vi "911 Vehicle Approach.vi"(3 "Cycle State In":T1) -> (0 "Cycle State Out":T1)   [LabVIEW 2020]
uses:
  Reset.ctl
  Cycle Status.ctl
  Cycle Enum.ctl
  Grade Gate.ctl
  Global Indicators.vi
panel:
  out "Cycle Status":T2
  in  "Reset":T3
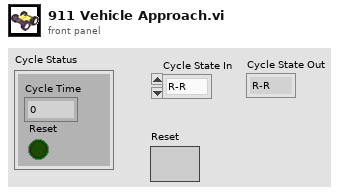
[diagram p1: front panel]
types:
  T1 = typedef "Cycle Enum.ctl" = enum16{"R-R", "NS Left G", "NS Left Y", "NS Straight G", "NS Straight Y", "r-r", "WE Left G", "WE Left Y", "WE Straight G", "WE Straight Y", "N All G", "S All G", "W All G", "E All G", "Gate Up", "Gate Mid", "Blink 1", "End Train", "Blink 2"}
  T2 = typedef "Cycle Status.ctl" = cluster{"Cycle Time":dbl, "Reset":bool}
  T3 = typedef "Reset.ctl" = bool
  T4 = typedef "Grade Gate.ctl" = cluster{"UP 2":bool, "Pivot":bool, "UP 3":bool, "UP 4":bool, "UP 5":bool, "UP 6":bool, "DOWN 2":bool, "DOWN 3":bool, "DOWN 4":bool, "DOWN 5":bool, "DOWN 6":bool, "DOWN 7":bool, "DOWN 8":bool, "SIDE 2":bool, "SIDE 3":bool, "SIDE 4":bool, "SIDE 5":bool, "Blinky 2":bool, "Blinky 1":bool}
  T5 = typedef "Traffic Signal.ctl" = cluster{"Red Light":bool, "Yellow Light":bool, "Green Light":bool, "Yellow Turn":bool, "Green Turn":bool}
  T6 = typedef "PedX Signal.ctl" = cluster{"PedX Walk":bool, "PedX Stop":bool}
  T7 = enum16{"R-R", "NS Left G", "NS Left Y", "NS Straight G", "NS Straight Y", "r-r", "WE Left G", "WE Left Y", "WE Straight G", "WE Straight Y"}
  T8 = enum16{"R-R", "NS Left G", "NS Left Y", "NS Straight G", "NS Straight Y"}
  T9 = cluster{"North":bool, "South":bool, "West":bool, "East":bool}
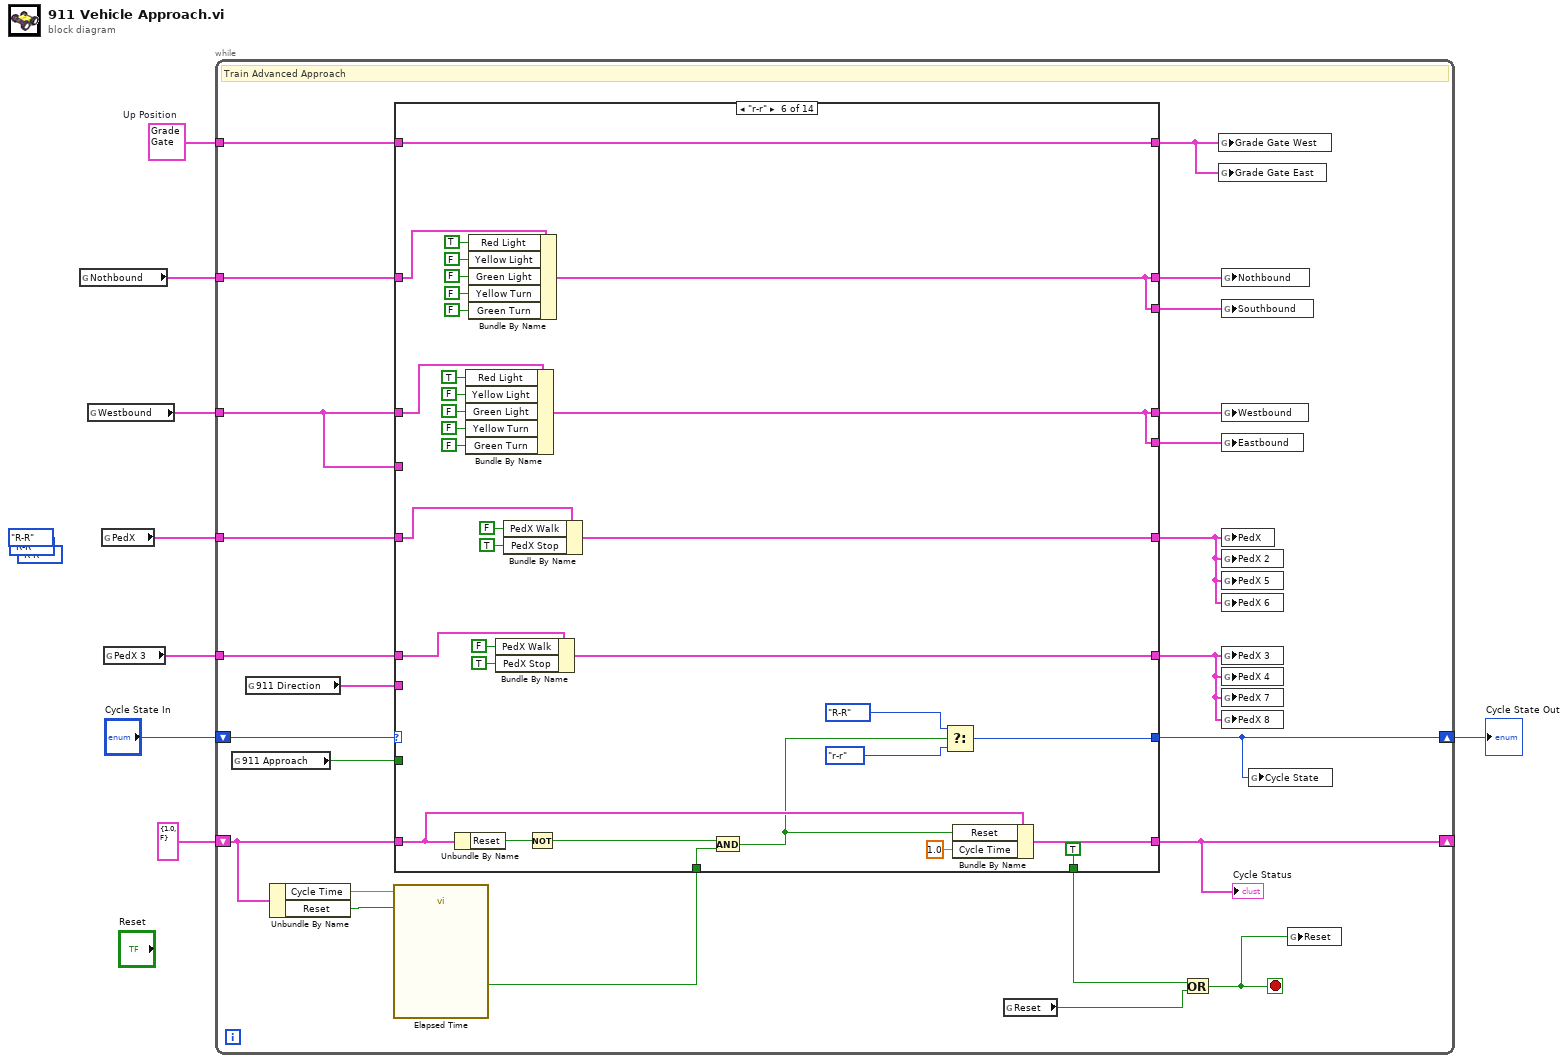
[diagram p0: block diagram]
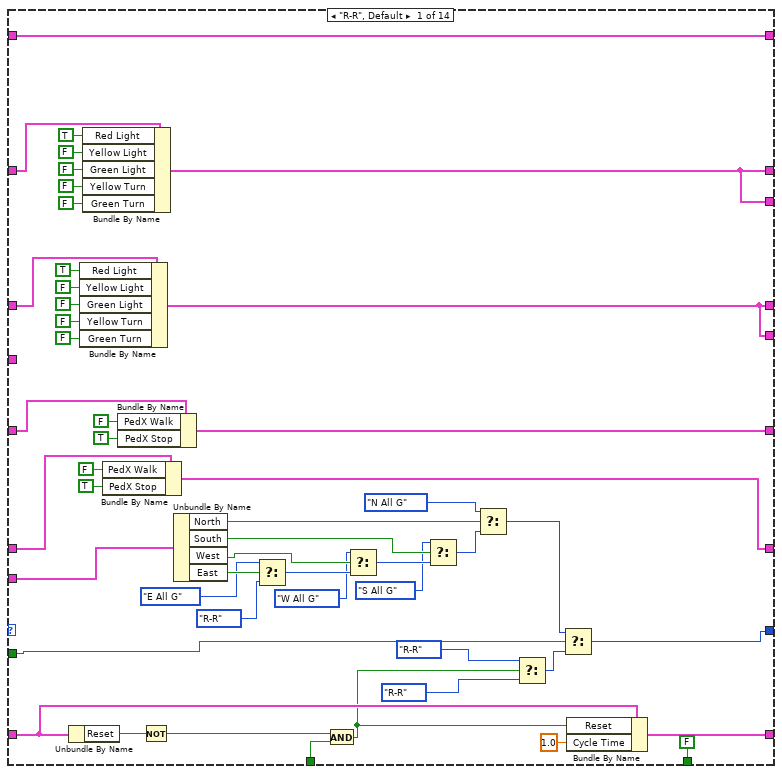
[diagram p2: hidden frame]
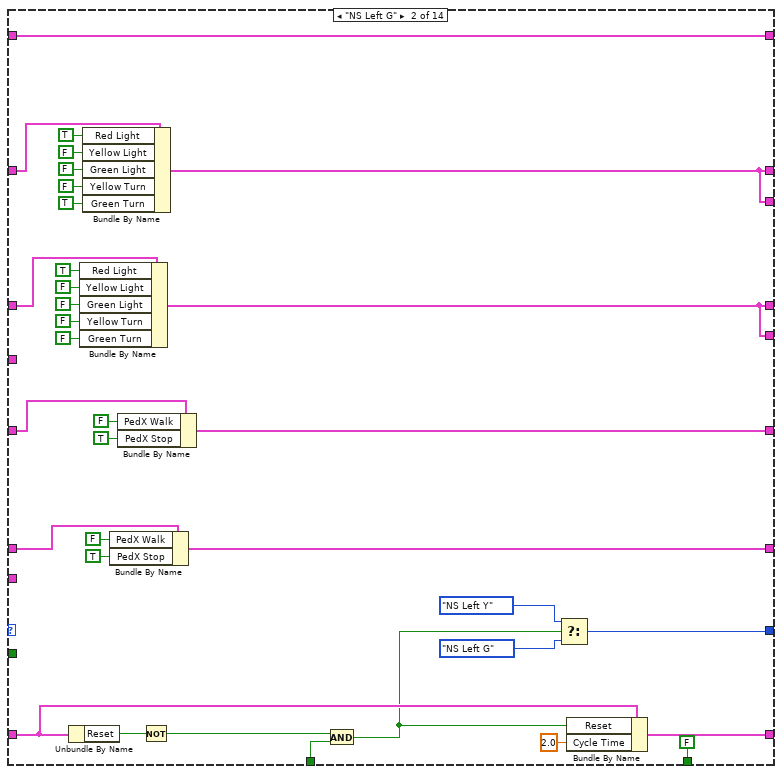
[diagram p3: hidden frame]
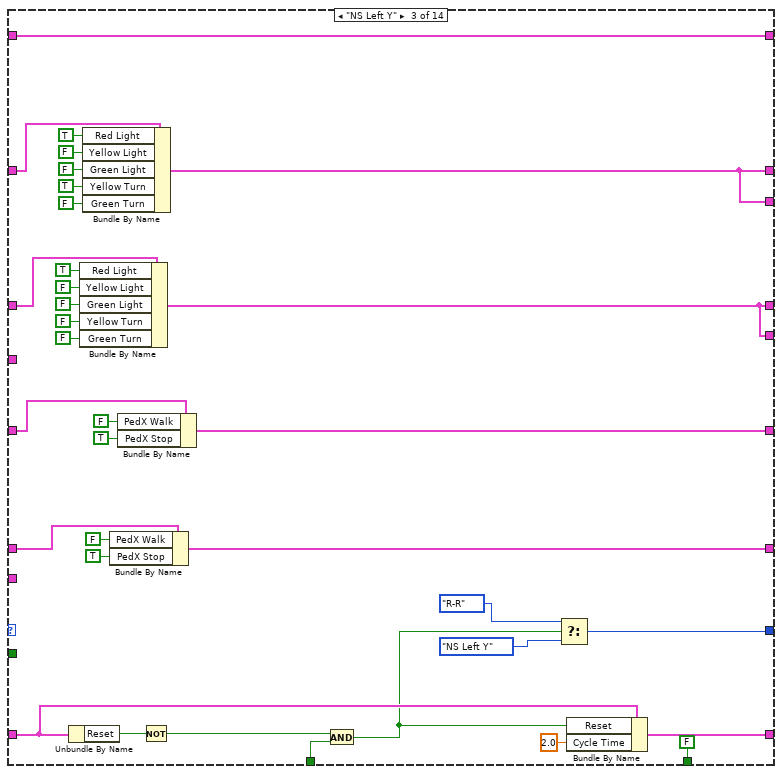
[diagram p4: hidden frame]
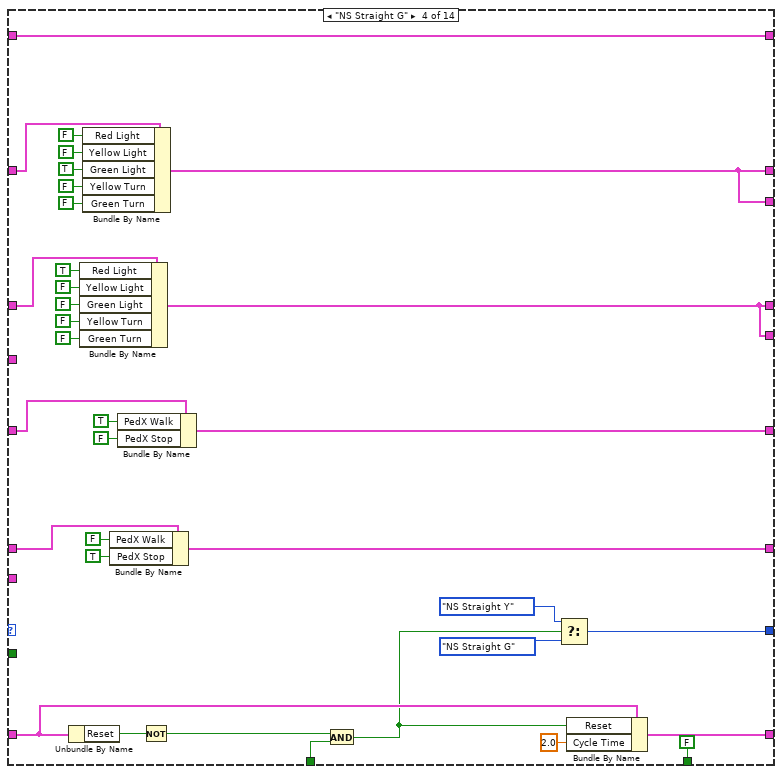
[diagram p5: hidden frame]
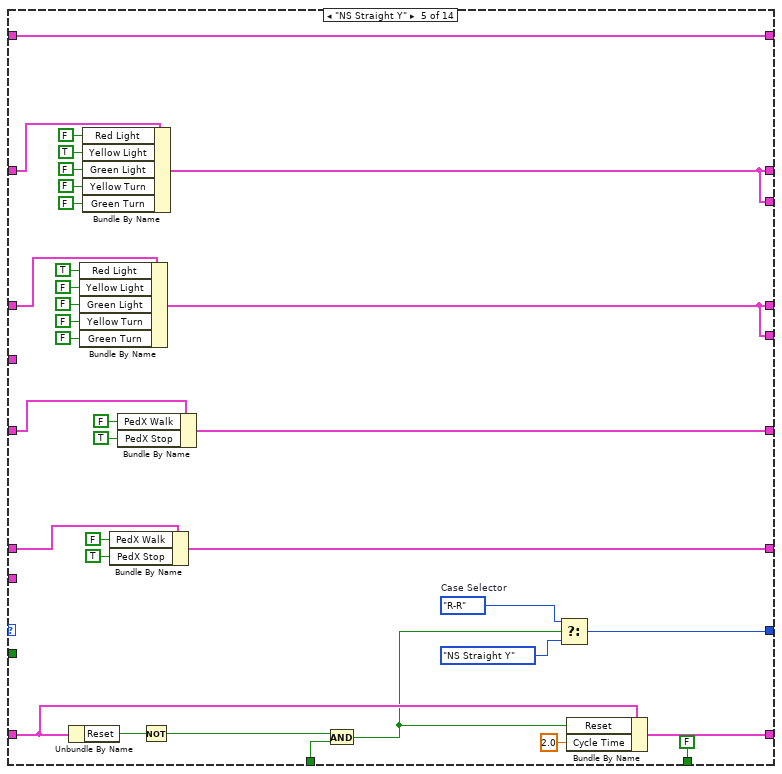
[diagram p6: hidden frame]
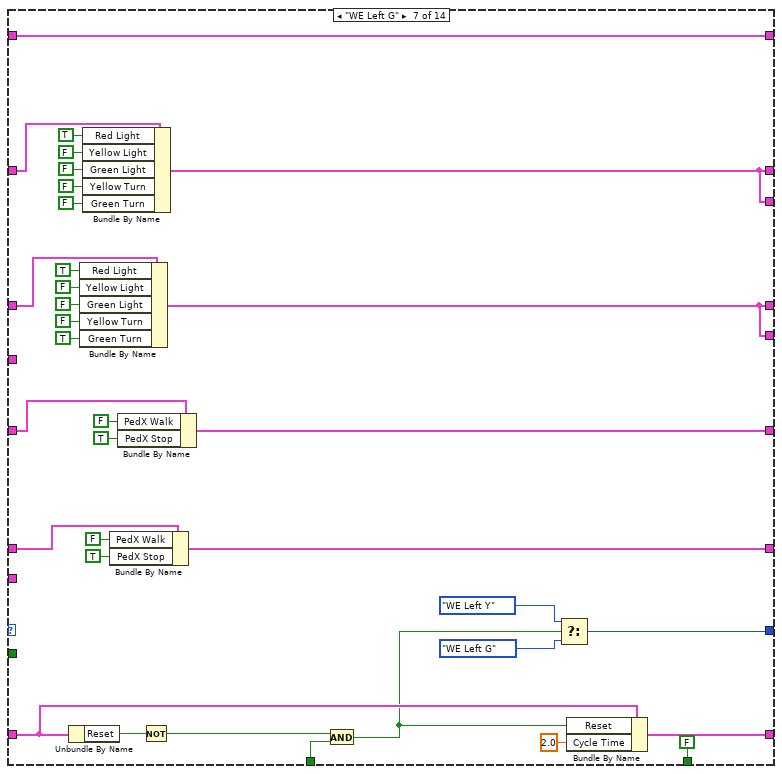
[diagram p7: hidden frame]
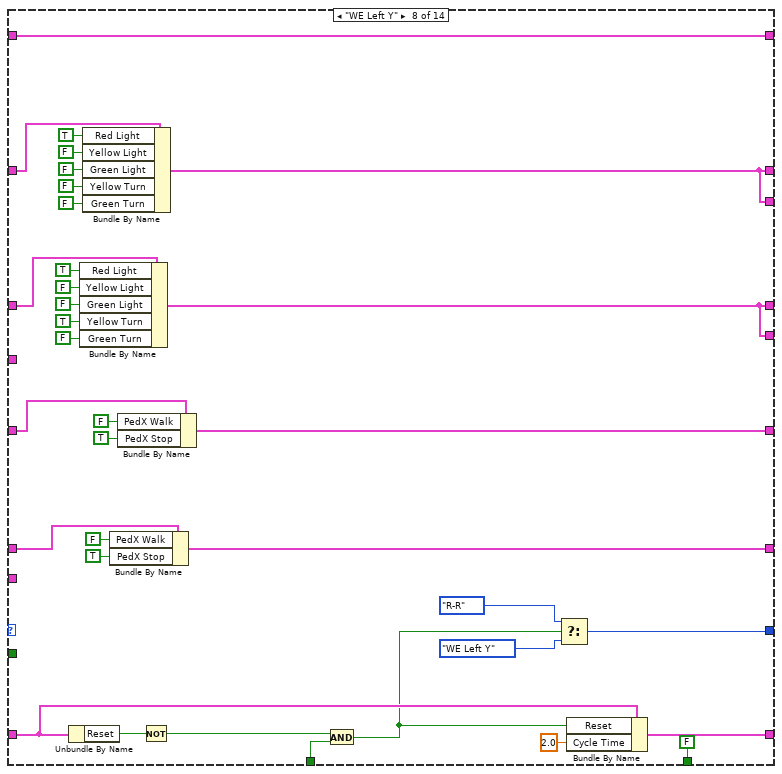
[diagram p8: hidden frame]
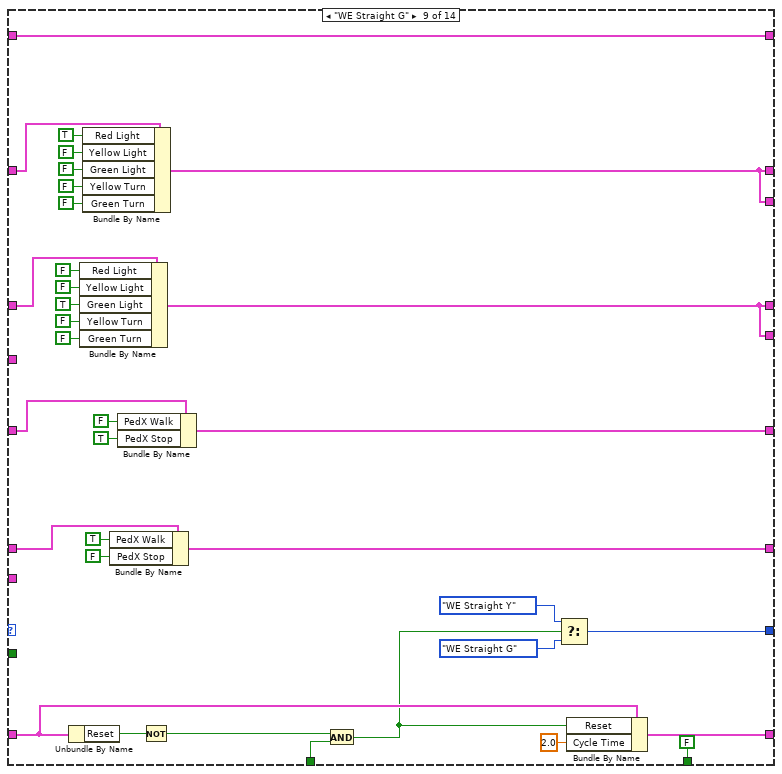
[diagram p9: hidden frame]
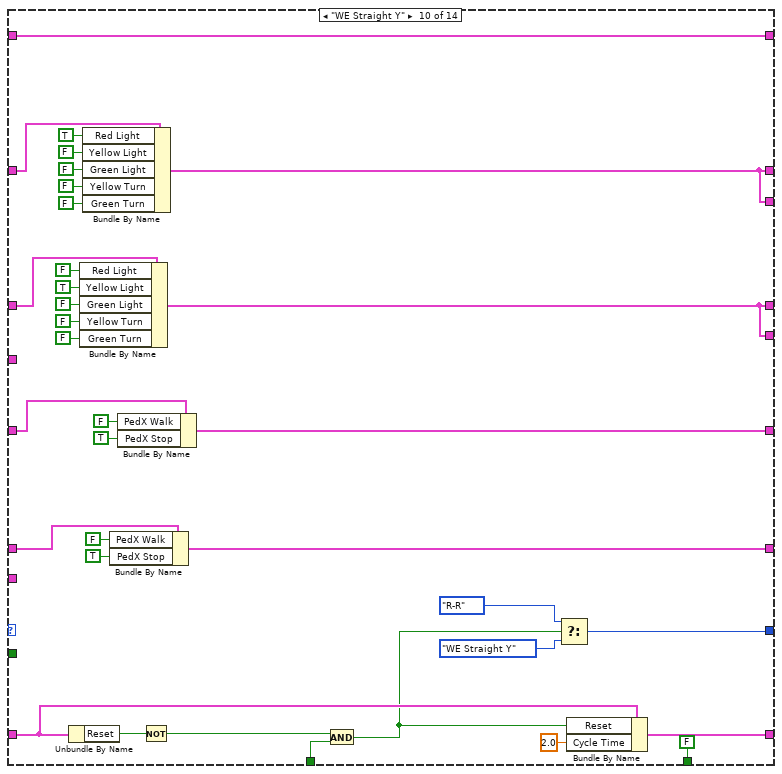
[diagram p10: hidden frame]
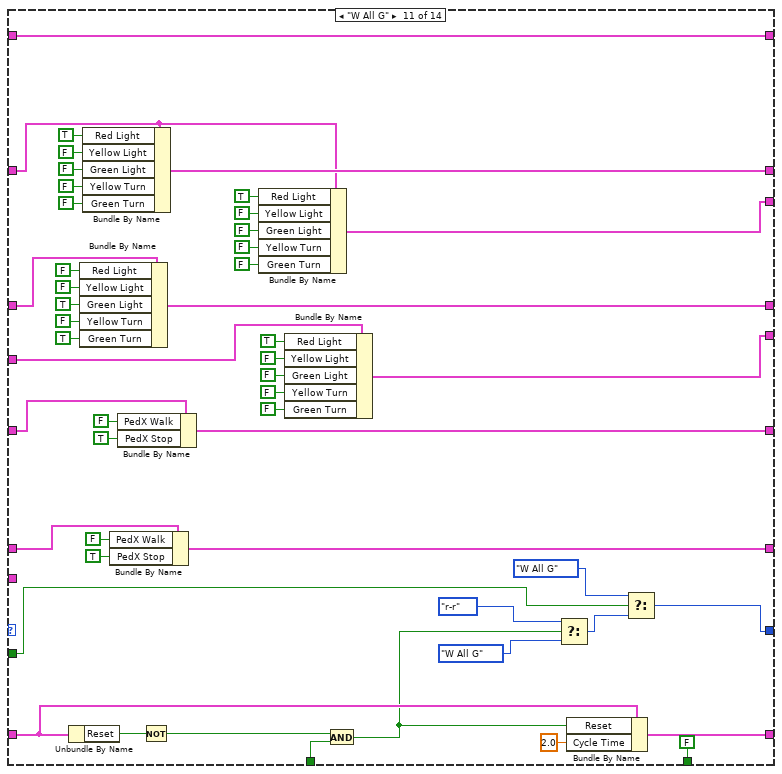
[diagram p11: hidden frame]
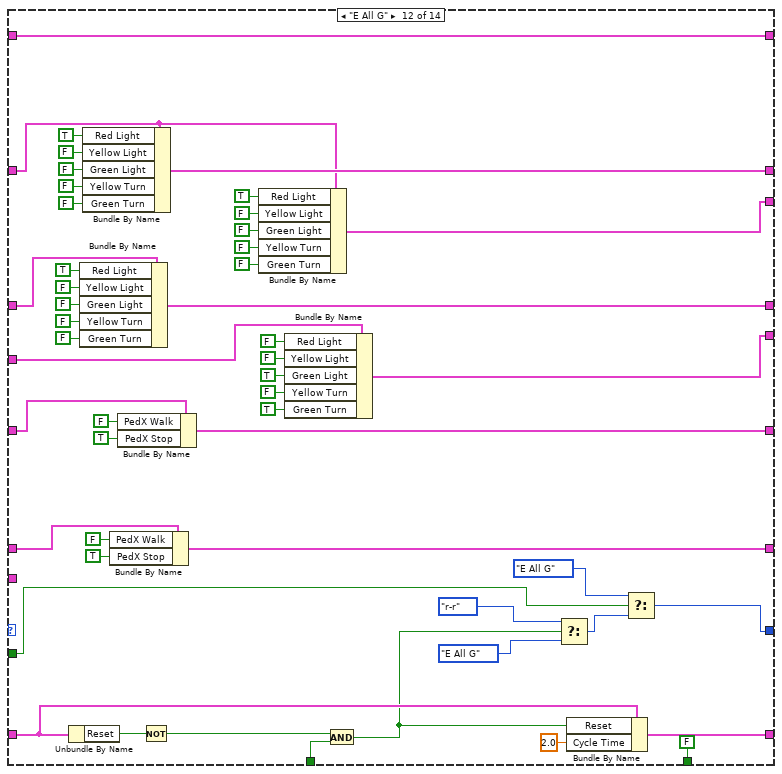
[diagram p12: hidden frame]
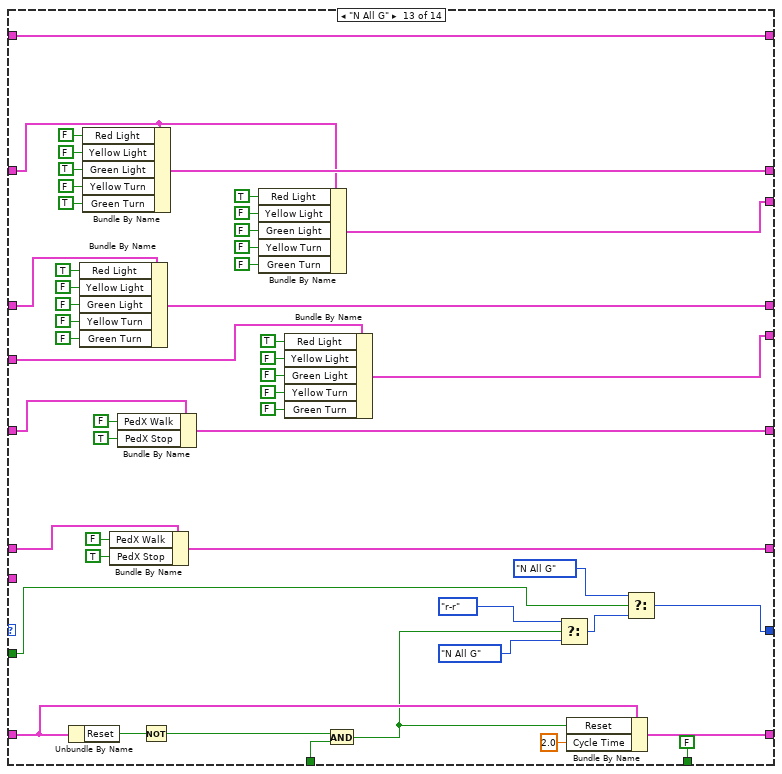
[diagram p13: hidden frame]
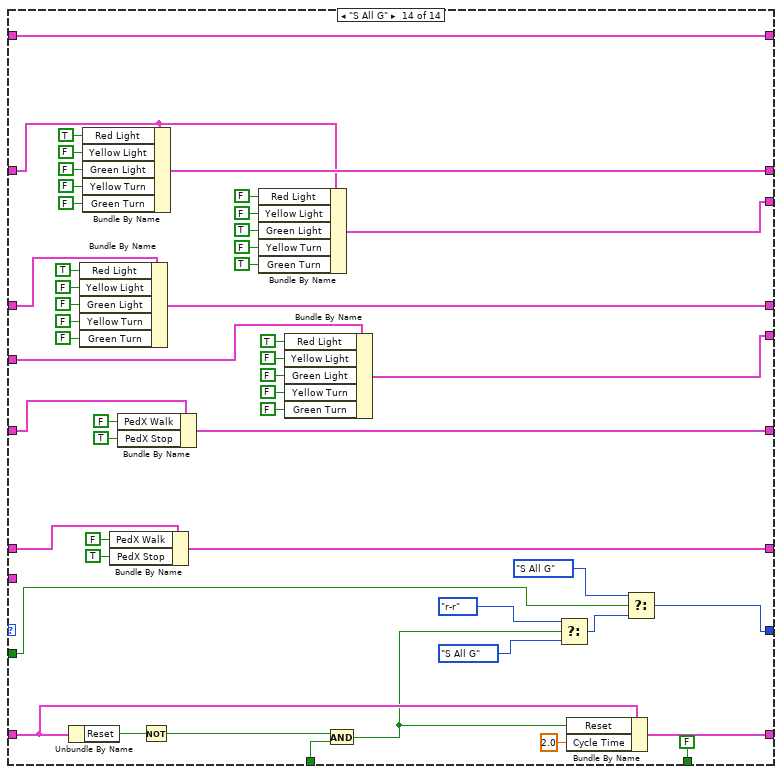
[diagram p14: hidden frame]
diagram:
  (unwired) Cycle_Enum."R-R" ("Cycle State In")
  (unwired) Cycle_Enum."R-R" ("Cycle State In")
  (unwired) Cycle_Enum."R-R" ("Cycle State In")
  w8 = T4 {"UP 2"=FALSE, "Pivot"=FALSE, "UP 3"=TRUE, "UP 4"=FALSE, "UP 5"=FALSE, "UP 6"=FALSE, "DOWN 2"=FALSE, "DOWN 3"=FALSE, "DOWN 4"=FALSE, "DOWN 5"=FALSE, "DOWN 6"=FALSE, "DOWN 7"=FALSE, "DOWN 8"=FALSE, "SIDE 2"=FALSE, "SIDE 3"=FALSE, "SIDE 4"=FALSE, "SIDE 5"=FALSE, "Blinky 2"=FALSE, "Blinky 1"=FALSE}  # Up Position
  n1 = global read "Global Indicators.vi" "Nothbound"() -> (w6:T5)
  n2 = global read "Global Indicators.vi" "Westbound"() -> (w5:T5)
  n3 = global read "Global Indicators.vi" "PedX"() -> (w4:T6)
  n4 = global read "Global Indicators.vi" "PedX 3"() -> (w3:T6)
  n5 = while {
    shift-right: [w17] -> w1
    shift-left: "Cycle State In" -> [w19]
    tunnel: w8 -> [w28]
    tunnel: w5 -> [w16]
    tunnel: w6 -> [w27]
    tunnel: w4 -> [w26]
    tunnel: w3 -> [w25]
    shift-right: [w18] -> _
    shift-left: T2 {"Cycle Time"=1.0, "Reset"=FALSE} ("Cycle Status") -> [w24]
    stop <- w11 stop-if-true
    # "Train Advanced Approach"
    n6 = global read "Global Indicators.vi" "911 Approach"() -> (w12:bool)
    n7 = global read "Global Indicators.vi" "911 Direction"() -> (w10:T9)
    n8 = Unbundle By Name(w24) -> ("Cycle Time"=w32:dbl, "Reset"=w31:bool)
    n9 = call "Elapsed Time"("Time Target (s)"=w32, "Reset"=w31) -> ("Time has Elapsed"=w30:bool)  [unwired: 10 in, 7 out]
    n10 = case shown="\"r-r\"" w19 {
      tunnel: [w82 w116 w150 w184 w218 w252 w286 w320 w354 w388 w438 w488 w538 w588] -> w29
      tunnel: w28 -> [w82 w116 w150 w184 w218 w252 w286 w320 w354 w388 w438 w488 w538 w588]
      tunnel: [w33 w83 w117 w151 w185 w219 w253 w287 w321 w355 w432 w482 w532 w582] -> w23
      tunnel: w27 -> [w81 w115 w149 w183 w217 w251 w285 w319 w353 w387 w395 w445 w495 w545]
      tunnel: [w53 w85 w119 w153 w187 w221 w255 w289 w323 w357 w419 w469 w519 w569] -> w22
      tunnel: w16 -> [w64 w97 w130 w163 w199 w233 w267 w301 w335 w369 w420 w470 w520 w570]
      tunnel: [w72 w106 w140 w174 w208 w242 w276 w310 w344 w378 w428 w478 w528 w578] -> w21
      tunnel: w26 -> [w75 w109 w143 w177 w211 w245 w279 w313 w347 w381 w431 w481 w531 w581]
      tunnel: w25 -> [w55 w88 w121 w154 w190 w224 w258 w292 w326 w360 w410 w460 w510 w560]
      tunnel: [w56 w89 w122 w155 w191 w225 w259 w293 w327 w361 w411 w461 w511 w561] -> w20
      tunnel: [w68 w101 w134 w167 w203 w237 w271 w305 w339 w373 w424 w474 w524 w574] -> w18
      tunnel: w24 -> [w67 w100 w133 w166 w202 w236 w270 w304 w338 w372 w423 w473 w523 w573]
      tunnel: [w49 w102 w136 w170 w204 w238 w272 w306 w340 w374 w396 w446 w496 w546] -> w17
      tunnel: w30 -> [w69 w103 w137 w171 w205 w239 w273 w307 w341 w375 w425 w475 w525 w575]
      tunnel: w16 -> [_ _ _ _ _ _ _ _ _ _ w409 w459 w509 w559]
      tunnel: [w53 w85 w119 w153 w187 w221 w255 w289 w323 w357 w403 w453 w503 w553] -> w15
      tunnel: w12 -> [w48 _ _ _ _ _ _ _ _ _ w399 w449 w499 w549]
      tunnel: [FALSE FALSE FALSE FALSE FALSE TRUE FALSE FALSE FALSE FALSE FALSE FALSE FALSE FALSE] -> w13
      tunnel: w10 -> [w47 _ _ _ _ _ _ _ _ _ _ _ _ _]
      tunnel: [w33 w83 w117 w151 w185 w219 w253 w287 w321 w355 w389 w439 w489 w539] -> w9
      frame "R-R", Default {
        n11 = Unbundle By Name(w67) -> ("Reset"=w71:bool)
        n12 = Bundle By Name(cluster=w64, "Red Light"=TRUE, "Yellow Light"=FALSE, "Green Light"=FALSE, "Yellow Turn"=FALSE, "Green Turn"=FALSE) -> (w53:T5)
        n13 = Bundle By Name(cluster=w81, "Red Light"=TRUE, "Yellow Light"=FALSE, "Green Light"=FALSE, "Yellow Turn"=FALSE, "Green Turn"=FALSE) -> (w33:T5)
        n14 = Bundle By Name(cluster=w55, "PedX Walk"=FALSE, "PedX Stop"=TRUE) -> (w56:T6)
        n15 = Bundle By Name(cluster=w75, "PedX Walk"=FALSE, "PedX Stop"=TRUE) -> (w72:T6)
        n16 = Not(x=w71) -> (.not. x?=w70:bool)
        n17 = Unbundle By Name(w47) -> ("North"=w46:bool, "South"=w38:bool, "West"=w42:bool, "East"=w45:bool)
        n18 = Select(t=Cycle_Enum."E All G" ("Cycle State In"), s=w45, f=Cycle_Enum."R-R" ("Cycle State In")) -> (s? t:f=w41:T1)
        n19 = And(x=w70, y=w69) -> (x .and. y?=w66:bool)
        n20 = Select(t=Cycle_Enum."W All G" ("Cycle State In"), s=w42, f=w41) -> (s? t:f=w39:T1)
        n21 = Select(t=Cycle_Enum."S All G" ("Cycle State In"), s=w38, f=w39) -> (s? t:f=w36:T1)
        n22 = Select(t=Cycle_Enum."N All G" ("Cycle State In"), s=w46, f=w36) -> (s? t:f=w34:T1)
        n23 = Select(t=Cycle_Enum."R-R" ("Cycle State In"), s=w66, f=Cycle_Enum."R-R" ("Cycle State In")) -> (s? t:f=w50:T1)
        n24 = Select(t=w34, s=w48, f=w50) -> (s? t:f=w49:T1)
        n25 = Bundle By Name(cluster=w67, "Reset"=w66, "Cycle Time"=1.0) -> (w68:T2)
      }
      frame "NS Left G" {
        n26 = Unbundle By Name(w100) -> ("Reset"=w105:bool)
        n27 = Bundle By Name(cluster=w97, "Red Light"=TRUE, "Yellow Light"=FALSE, "Green Light"=FALSE, "Yellow Turn"=FALSE, "Green Turn"=FALSE) -> (w85:T5)
        n28 = Bundle By Name(cluster=w115, "Red Light"=TRUE, "Yellow Light"=FALSE, "Green Light"=FALSE, "Yellow Turn"=FALSE, "Green Turn"=TRUE) -> (w83:T5)
        n29 = Bundle By Name(cluster=w88, "PedX Walk"=FALSE, "PedX Stop"=TRUE) -> (w89:T6)
        n30 = Bundle By Name(cluster=w109, "PedX Walk"=FALSE, "PedX Stop"=TRUE) -> (w106:T6)
        n31 = Not(x=w105) -> (.not. x?=w104:bool)
        n32 = And(x=w104, y=w103) -> (x .and. y?=w99:bool)
        n33 = Select(t=T7."NS Left Y" ("Case Selector"), s=w99, f=T7."NS Left G" ("Case Selector")) -> (s? t:f=w102:T7)
        n34 = Bundle By Name(cluster=w100, "Reset"=w99, "Cycle Time"=2.0) -> (w101:T2)
      }
      frame "NS Left Y" {
        n35 = Unbundle By Name(w133) -> ("Reset"=w139:bool)
        n36 = Bundle By Name(cluster=w130, "Red Light"=TRUE, "Yellow Light"=FALSE, "Green Light"=FALSE, "Yellow Turn"=FALSE, "Green Turn"=FALSE) -> (w119:T5)
        n37 = Bundle By Name(cluster=w149, "Red Light"=TRUE, "Yellow Light"=FALSE, "Green Light"=FALSE, "Yellow Turn"=TRUE, "Green Turn"=FALSE) -> (w117:T5)
        n38 = Bundle By Name(cluster=w121, "PedX Walk"=FALSE, "PedX Stop"=TRUE) -> (w122:T6)
        n39 = Bundle By Name(cluster=w143, "PedX Walk"=FALSE, "PedX Stop"=TRUE) -> (w140:T6)
        n40 = Not(x=w139) -> (.not. x?=w138:bool)
        n41 = And(x=w138, y=w137) -> (x .and. y?=w132:bool)
        n42 = Select(t=Cycle_Enum."R-R" ("Cycle State In"), s=w132, f=T8."NS Left Y" ("Case Selector")) -> (s? t:f=w136:T1)
        n43 = Bundle By Name(cluster=w133, "Reset"=w132, "Cycle Time"=2.0) -> (w134:T2)
      }
      frame "NS Straight G" {
        n44 = Unbundle By Name(w166) -> ("Reset"=w173:bool)
        n45 = Bundle By Name(cluster=w163, "Red Light"=TRUE, "Yellow Light"=FALSE, "Green Light"=FALSE, "Yellow Turn"=FALSE, "Green Turn"=FALSE) -> (w153:T5)
        n46 = Bundle By Name(cluster=w183, "Red Light"=FALSE, "Yellow Light"=FALSE, "Green Light"=TRUE, "Yellow Turn"=FALSE, "Green Turn"=FALSE) -> (w151:T5)
        n47 = Bundle By Name(cluster=w154, "PedX Walk"=FALSE, "PedX Stop"=TRUE) -> (w155:T6)
        n48 = Bundle By Name(cluster=w177, "PedX Walk"=TRUE, "PedX Stop"=FALSE) -> (w174:T6)
        n49 = Not(x=w173) -> (.not. x?=w172:bool)
        n50 = And(x=w172, y=w171) -> (x .and. y?=w165:bool)
        n51 = Select(t=T8."NS Straight Y" ("Case Selector"), s=w165, f=T8."NS Straight G" ("Case Selector")) -> (s? t:f=w170:T8)
        n52 = Bundle By Name(cluster=w166, "Reset"=w165, "Cycle Time"=2.0) -> (w167:T2)
      }
      frame "NS Straight Y" {
        w189 = T7."R-R"  # Case Selector
        n53 = Unbundle By Name(w202) -> ("Reset"=w207:bool)
        n54 = Bundle By Name(cluster=w199, "Red Light"=TRUE, "Yellow Light"=FALSE, "Green Light"=FALSE, "Yellow Turn"=FALSE, "Green Turn"=FALSE) -> (w187:T5)
        n55 = Bundle By Name(cluster=w217, "Red Light"=FALSE, "Yellow Light"=TRUE, "Green Light"=FALSE, "Yellow Turn"=FALSE, "Green Turn"=FALSE) -> (w185:T5)
        n56 = Bundle By Name(cluster=w190, "PedX Walk"=FALSE, "PedX Stop"=TRUE) -> (w191:T6)
        n57 = Bundle By Name(cluster=w211, "PedX Walk"=FALSE, "PedX Stop"=TRUE) -> (w208:T6)
        n58 = Not(x=w207) -> (.not. x?=w206:bool)
        n59 = And(x=w206, y=w205) -> (x .and. y?=w201:bool)
        n60 = Select(t=w189, s=w201, f=T7."NS Straight Y" ("Case Selector")) -> (s? t:f=w204:T7)
        n61 = Bundle By Name(cluster=w202, "Reset"=w201, "Cycle Time"=2.0) -> (w203:T2)
      }
      frame "r-r" {
        n62 = Unbundle By Name(w236) -> ("Reset"=w241:bool)
        n63 = Bundle By Name(cluster=w233, "Red Light"=TRUE, "Yellow Light"=FALSE, "Green Light"=FALSE, "Yellow Turn"=FALSE, "Green Turn"=FALSE) -> (w221:T5)
        n64 = Bundle By Name(cluster=w251, "Red Light"=TRUE, "Yellow Light"=FALSE, "Green Light"=FALSE, "Yellow Turn"=FALSE, "Green Turn"=FALSE) -> (w219:T5)
        n65 = Bundle By Name(cluster=w224, "PedX Walk"=FALSE, "PedX Stop"=TRUE) -> (w225:T6)
        n66 = Bundle By Name(cluster=w245, "PedX Walk"=FALSE, "PedX Stop"=TRUE) -> (w242:T6)
        n67 = Not(x=w241) -> (.not. x?=w240:bool)
        n68 = And(x=w240, y=w239) -> (x .and. y?=w235:bool)
        n69 = Select(t=T7."R-R" ("Case Selector"), s=w235, f=T7."r-r" ("Case Selector")) -> (s? t:f=w238:T7)
        n70 = Bundle By Name(cluster=w236, "Reset"=w235, "Cycle Time"=1.0) -> (w237:T2)
      }
      frame "WE Left G" {
        n71 = Unbundle By Name(w270) -> ("Reset"=w275:bool)
        n72 = Bundle By Name(cluster=w267, "Red Light"=TRUE, "Yellow Light"=FALSE, "Green Light"=FALSE, "Yellow Turn"=FALSE, "Green Turn"=TRUE) -> (w255:T5)
        n73 = Bundle By Name(cluster=w285, "Red Light"=TRUE, "Yellow Light"=FALSE, "Green Light"=FALSE, "Yellow Turn"=FALSE, "Green Turn"=FALSE) -> (w253:T5)
        n74 = Bundle By Name(cluster=w258, "PedX Walk"=FALSE, "PedX Stop"=TRUE) -> (w259:T6)
        n75 = Bundle By Name(cluster=w279, "PedX Walk"=FALSE, "PedX Stop"=TRUE) -> (w276:T6)
        n76 = Not(x=w275) -> (.not. x?=w274:bool)
        n77 = And(x=w274, y=w273) -> (x .and. y?=w269:bool)
        n78 = Select(t=T7."WE Left Y" ("Case Selector"), s=w269, f=T7."WE Left G" ("Case Selector")) -> (s? t:f=w272:T7)
        n79 = Bundle By Name(cluster=w270, "Reset"=w269, "Cycle Time"=2.0) -> (w271:T2)
      }
      frame "WE Left Y" {
        n80 = Unbundle By Name(w304) -> ("Reset"=w309:bool)
        n81 = Bundle By Name(cluster=w301, "Red Light"=TRUE, "Yellow Light"=FALSE, "Green Light"=FALSE, "Yellow Turn"=TRUE, "Green Turn"=FALSE) -> (w289:T5)
        n82 = Bundle By Name(cluster=w319, "Red Light"=TRUE, "Yellow Light"=FALSE, "Green Light"=FALSE, "Yellow Turn"=FALSE, "Green Turn"=FALSE) -> (w287:T5)
        n83 = Bundle By Name(cluster=w292, "PedX Walk"=FALSE, "PedX Stop"=TRUE) -> (w293:T6)
        n84 = Bundle By Name(cluster=w313, "PedX Walk"=FALSE, "PedX Stop"=TRUE) -> (w310:T6)
        n85 = Not(x=w309) -> (.not. x?=w308:bool)
        n86 = And(x=w308, y=w307) -> (x .and. y?=w303:bool)
        n87 = Select(t=T7."R-R" ("Case Selector"), s=w303, f=T7."WE Left Y" ("Case Selector")) -> (s? t:f=w306:T7)
        n88 = Bundle By Name(cluster=w304, "Reset"=w303, "Cycle Time"=2.0) -> (w305:T2)
      }
      frame "WE Straight G" {
        n89 = Unbundle By Name(w338) -> ("Reset"=w343:bool)
        n90 = Bundle By Name(cluster=w335, "Red Light"=FALSE, "Yellow Light"=FALSE, "Green Light"=TRUE, "Yellow Turn"=FALSE, "Green Turn"=FALSE) -> (w323:T5)
        n91 = Bundle By Name(cluster=w353, "Red Light"=TRUE, "Yellow Light"=FALSE, "Green Light"=FALSE, "Yellow Turn"=FALSE, "Green Turn"=FALSE) -> (w321:T5)
        n92 = Bundle By Name(cluster=w326, "PedX Walk"=TRUE, "PedX Stop"=FALSE) -> (w327:T6)
        n93 = Bundle By Name(cluster=w347, "PedX Walk"=FALSE, "PedX Stop"=TRUE) -> (w344:T6)
        n94 = Not(x=w343) -> (.not. x?=w342:bool)
        n95 = And(x=w342, y=w341) -> (x .and. y?=w337:bool)
        n96 = Select(t=T7."WE Straight Y" ("Case Selector"), s=w337, f=T7."WE Straight G" ("Case Selector")) -> (s? t:f=w340:T7)
        n97 = Bundle By Name(cluster=w338, "Reset"=w337, "Cycle Time"=2.0) -> (w339:T2)
      }
      frame "WE Straight Y" {
        n98 = Unbundle By Name(w372) -> ("Reset"=w377:bool)
        n99 = Bundle By Name(cluster=w369, "Red Light"=FALSE, "Yellow Light"=TRUE, "Green Light"=FALSE, "Yellow Turn"=FALSE, "Green Turn"=FALSE) -> (w357:T5)
        n100 = Bundle By Name(cluster=w387, "Red Light"=TRUE, "Yellow Light"=FALSE, "Green Light"=FALSE, "Yellow Turn"=FALSE, "Green Turn"=FALSE) -> (w355:T5)
        n101 = Bundle By Name(cluster=w360, "PedX Walk"=FALSE, "PedX Stop"=TRUE) -> (w361:T6)
        n102 = Bundle By Name(cluster=w381, "PedX Walk"=FALSE, "PedX Stop"=TRUE) -> (w378:T6)
        n103 = Not(x=w377) -> (.not. x?=w376:bool)
        n104 = And(x=w376, y=w375) -> (x .and. y?=w371:bool)
        n105 = Select(t=T7."R-R" ("Case Selector"), s=w371, f=T7."WE Straight Y" ("Case Selector")) -> (s? t:f=w374:T7)
        n106 = Bundle By Name(cluster=w372, "Reset"=w371, "Cycle Time"=2.0) -> (w373:T2)
      }
      frame "W All G" {
        n107 = Unbundle By Name(w423) -> ("Reset"=w427:bool)
        n108 = Bundle By Name(cluster=w420, "Red Light"=FALSE, "Yellow Light"=FALSE, "Green Light"=TRUE, "Yellow Turn"=FALSE, "Green Turn"=TRUE) -> (w419:T5)
        n109 = Bundle By Name(cluster=w395, "Red Light"=TRUE, "Yellow Light"=FALSE, "Green Light"=FALSE, "Yellow Turn"=FALSE, "Green Turn"=FALSE) -> (w432:T5)
        n110 = Bundle By Name(cluster=w410, "PedX Walk"=FALSE, "PedX Stop"=TRUE) -> (w411:T6)
        n111 = Bundle By Name(cluster=w431, "PedX Walk"=FALSE, "PedX Stop"=TRUE) -> (w428:T6)
        n112 = Not(x=w427) -> (.not. x?=w426:bool)
        n113 = Bundle By Name(cluster=w395, "Red Light"=TRUE, "Yellow Light"=FALSE, "Green Light"=FALSE, "Yellow Turn"=FALSE, "Green Turn"=FALSE) -> (w389:T5)
        n114 = Bundle By Name(cluster=w409, "Red Light"=TRUE, "Yellow Light"=FALSE, "Green Light"=FALSE, "Yellow Turn"=FALSE, "Green Turn"=FALSE) -> (w403:T5)
        n115 = And(x=w426, y=w425) -> (x .and. y?=w422:bool)
        n116 = Select(t=Cycle_Enum."r-r" ("Cycle State In"), s=w422, f=Cycle_Enum."W All G" ("Cycle State In")) -> (s? t:f=w398:T1)
        n117 = Bundle By Name(cluster=w423, "Reset"=w422, "Cycle Time"=2.0) -> (w424:T2)
        n118 = Select(t=Cycle_Enum."W All G" ("Cycle State In"), s=w399, f=w398) -> (s? t:f=w396:T1)
      }
      frame "E All G" {
        n119 = Unbundle By Name(w473) -> ("Reset"=w477:bool)
        n120 = Bundle By Name(cluster=w470, "Red Light"=TRUE, "Yellow Light"=FALSE, "Green Light"=FALSE, "Yellow Turn"=FALSE, "Green Turn"=FALSE) -> (w469:T5)
        n121 = Bundle By Name(cluster=w445, "Red Light"=TRUE, "Yellow Light"=FALSE, "Green Light"=FALSE, "Yellow Turn"=FALSE, "Green Turn"=FALSE) -> (w482:T5)
        n122 = Bundle By Name(cluster=w460, "PedX Walk"=FALSE, "PedX Stop"=TRUE) -> (w461:T6)
        n123 = Bundle By Name(cluster=w481, "PedX Walk"=FALSE, "PedX Stop"=TRUE) -> (w478:T6)
        n124 = Not(x=w477) -> (.not. x?=w476:bool)
        n125 = Bundle By Name(cluster=w445, "Red Light"=TRUE, "Yellow Light"=FALSE, "Green Light"=FALSE, "Yellow Turn"=FALSE, "Green Turn"=FALSE) -> (w439:T5)
        n126 = Bundle By Name(cluster=w459, "Red Light"=FALSE, "Yellow Light"=FALSE, "Green Light"=TRUE, "Yellow Turn"=FALSE, "Green Turn"=TRUE) -> (w453:T5)
        n127 = And(x=w476, y=w475) -> (x .and. y?=w472:bool)
        n128 = Select(t=Cycle_Enum."r-r" ("Cycle State In"), s=w472, f=Cycle_Enum."E All G" ("Cycle State In")) -> (s? t:f=w448:T1)
        n129 = Bundle By Name(cluster=w473, "Reset"=w472, "Cycle Time"=2.0) -> (w474:T2)
        n130 = Select(t=Cycle_Enum."E All G" ("Cycle State In"), s=w449, f=w448) -> (s? t:f=w446:T1)
      }
      frame "N All G" {
        n131 = Unbundle By Name(w523) -> ("Reset"=w527:bool)
        n132 = Bundle By Name(cluster=w520, "Red Light"=TRUE, "Yellow Light"=FALSE, "Green Light"=FALSE, "Yellow Turn"=FALSE, "Green Turn"=FALSE) -> (w519:T5)
        n133 = Bundle By Name(cluster=w495, "Red Light"=FALSE, "Yellow Light"=FALSE, "Green Light"=TRUE, "Yellow Turn"=FALSE, "Green Turn"=TRUE) -> (w532:T5)
        n134 = Bundle By Name(cluster=w510, "PedX Walk"=FALSE, "PedX Stop"=TRUE) -> (w511:T6)
        n135 = Bundle By Name(cluster=w531, "PedX Walk"=FALSE, "PedX Stop"=TRUE) -> (w528:T6)
        n136 = Not(x=w527) -> (.not. x?=w526:bool)
        n137 = Bundle By Name(cluster=w495, "Red Light"=TRUE, "Yellow Light"=FALSE, "Green Light"=FALSE, "Yellow Turn"=FALSE, "Green Turn"=FALSE) -> (w489:T5)
        n138 = Bundle By Name(cluster=w509, "Red Light"=TRUE, "Yellow Light"=FALSE, "Green Light"=FALSE, "Yellow Turn"=FALSE, "Green Turn"=FALSE) -> (w503:T5)
        n139 = And(x=w526, y=w525) -> (x .and. y?=w522:bool)
        n140 = Select(t=Cycle_Enum."r-r" ("Cycle State In"), s=w522, f=Cycle_Enum."N All G" ("Cycle State In")) -> (s? t:f=w498:T1)
        n141 = Bundle By Name(cluster=w523, "Reset"=w522, "Cycle Time"=2.0) -> (w524:T2)
        n142 = Select(t=Cycle_Enum."N All G" ("Cycle State In"), s=w499, f=w498) -> (s? t:f=w496:T1)
      }
      frame "S All G" {
        n143 = Unbundle By Name(w573) -> ("Reset"=w577:bool)
        n144 = Bundle By Name(cluster=w570, "Red Light"=TRUE, "Yellow Light"=FALSE, "Green Light"=FALSE, "Yellow Turn"=FALSE, "Green Turn"=FALSE) -> (w569:T5)
        n145 = Bundle By Name(cluster=w545, "Red Light"=TRUE, "Yellow Light"=FALSE, "Green Light"=FALSE, "Yellow Turn"=FALSE, "Green Turn"=FALSE) -> (w582:T5)
        n146 = Bundle By Name(cluster=w560, "PedX Walk"=FALSE, "PedX Stop"=TRUE) -> (w561:T6)
        n147 = Bundle By Name(cluster=w581, "PedX Walk"=FALSE, "PedX Stop"=TRUE) -> (w578:T6)
        n148 = Not(x=w577) -> (.not. x?=w576:bool)
        n149 = Bundle By Name(cluster=w545, "Red Light"=FALSE, "Yellow Light"=FALSE, "Green Light"=TRUE, "Yellow Turn"=FALSE, "Green Turn"=TRUE) -> (w539:T5)
        n150 = Bundle By Name(cluster=w559, "Red Light"=TRUE, "Yellow Light"=FALSE, "Green Light"=FALSE, "Yellow Turn"=FALSE, "Green Turn"=FALSE) -> (w553:T5)
        n151 = And(x=w576, y=w575) -> (x .and. y?=w572:bool)
        n152 = Select(t=Cycle_Enum."r-r" ("Cycle State In"), s=w572, f=Cycle_Enum."S All G" ("Cycle State In")) -> (s? t:f=w548:T1)
        n153 = Bundle By Name(cluster=w573, "Reset"=w572, "Cycle Time"=2.0) -> (w574:T2)
        n154 = Select(t=Cycle_Enum."S All G" ("Cycle State In"), s=w549, f=w548) -> (s? t:f=w546:T1)
      }
    }
    "Cycle Status" <- w18
    n155 = global read "Global Indicators.vi" "Reset"() -> (w14:T3)
    n156 = Or(x=w13, y=w14) -> (x .or. y?=w11:T3)
    n157 = global write "Global Indicators.vi" "Grade Gate West"(w29) -> ()
    n158 = global write "Global Indicators.vi" "Grade Gate East"(w29) -> ()
    n159 = global write "Global Indicators.vi" "Nothbound"(w23) -> ()
    n160 = global write "Global Indicators.vi" "Southbound"(w9) -> ()
    n161 = global write "Global Indicators.vi" "Westbound"(w22) -> ()
    n162 = global write "Global Indicators.vi" "Eastbound"(w15) -> ()
    n163 = global write "Global Indicators.vi" "PedX"(w21) -> ()
    n164 = global write "Global Indicators.vi" "PedX 2"(w21) -> ()
    n165 = global write "Global Indicators.vi" "PedX 5"(w21) -> ()
    n166 = global write "Global Indicators.vi" "PedX 6"(w21) -> ()
    n167 = global write "Global Indicators.vi" "PedX 3"(w20) -> ()
    n168 = global write "Global Indicators.vi" "PedX 4"(w20) -> ()
    n169 = global write "Global Indicators.vi" "PedX 7"(w20) -> ()
    n170 = global write "Global Indicators.vi" "PedX 8"(w20) -> ()
    n171 = global write "Global Indicators.vi" "Cycle State"(w17) -> ()
    n172 = global write "Global Indicators.vi" "Reset"(w11) -> ()
  }
  "Cycle State Out" <- w1
